vi "Set Mode.vi"(8 "error in (no error)":errorcluster, 11 "Instrument in":refnum<class "Instrument.lvclass">) -> (0 "error out":errorcluster, 3 "Instrument out":refnum<class "Instrument.lvclass">)   [LabVIEW 2018, in "Instrument.lvclass"]
uses:
  Instrument.lvclass
  Instrument.lvclass/Instrument.ctl
  Device/Optics/Optics.lvclass/Optics.ctl
  Device/Optics/Opt_Selector/Opt_Selector.lvclass
  C:/Users/devstaff/sparc4/s4gui/Versao ZeroMQ REQ-REP/SPARC4_GUI -20241030/Device/Optics/Optics.lvclass
  Device/Optics/Opt_Continuous/Opt_Continuous.lvclass
  Server/Server.lvclass
  Device/Optics/Optics.lvclass
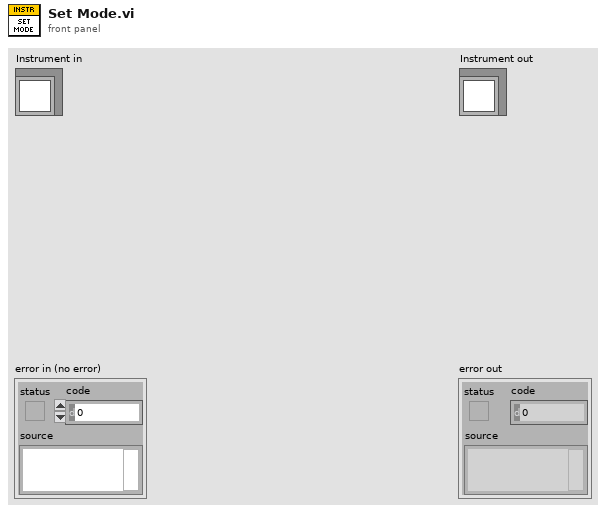
[diagram p1: front panel]
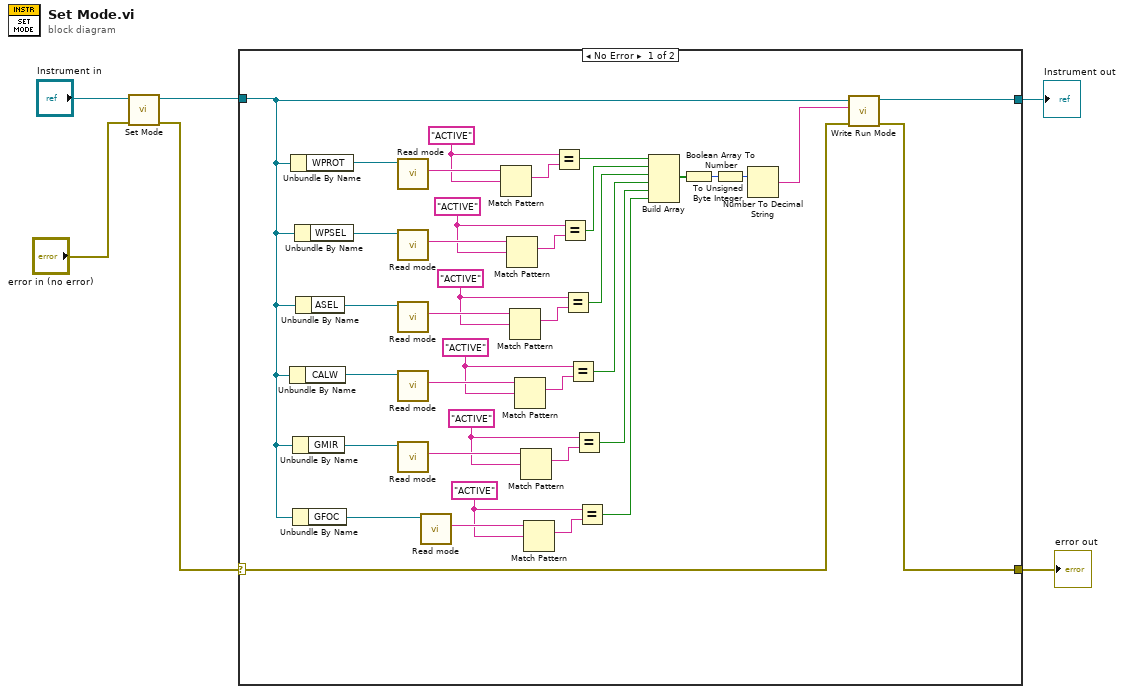
[diagram p0: block diagram]
diagram:
  n1 = call-parent "Set Mode.vi"("error in (no error)"="error in (no error)", "Server in"="Instrument in") -> ("error out"=w4:errorcluster, "Server out"=w3:refnum<class "Instrument.lvclass">)  [unwired: 8 in]
  n2 = case shown="No Error" w4 {
    selector: w4 -> [w18 w45]
    tunnel: w3 -> [w20 w46]
    tunnel: [w19 w46] -> w2
    tunnel: [w17 w45] -> w1
    frame No Error {
      w22 = "ACTIVE"
      w26 = "ACTIVE"
      w29 = "ACTIVE"
      w34 = "ACTIVE"
      w38 = "ACTIVE"
      w41 = "ACTIVE"
      n3 = Unbundle By Name(w20) -> ("CALW"=w32:refnum<class "Opt_Selector.lvclass">)
      n4 = Unbundle By Name(w20) -> ("WPROT"=w44:refnum<class "Opt_Selector.lvclass">)
      n5 = Unbundle By Name(w20) -> ("GMIR"=w25:refnum<class "Opt_Continuous.lvclass">)
      n6 = Unbundle By Name(w20) -> ("GFOC"=w21:refnum<class "Opt_Continuous.lvclass">)
      n7 = Unbundle By Name(w20) -> ("WPSEL"=w37:refnum<class "Opt_Selector.lvclass">)
      n8 = Unbundle By Name(w20) -> ("ASEL"=w33:refnum<class "Opt_Selector.lvclass">)
      n9 = call "Read mode.vi"("Optics in"=w44) -> ("mode"=w43:string)  [unwired: 8 in, 2 out]
      n10 = call "Read mode.vi"("Optics in"=w37) -> ("mode"=w40:string)  [unwired: 8 in, 2 out]
      n11 = call "Read mode.vi"("Optics in"=w33) -> ("mode"=w36:string)  [unwired: 8 in, 2 out]
      n12 = call "Read mode.vi"("Optics in"=w32) -> ("mode"=w31:string)  [unwired: 8 in, 2 out]
      n13 = call "Read mode.vi"("Optics in"=w25) -> ("mode"=w28:string)  [unwired: 8 in, 2 out]
      n14 = call "Read mode.vi"("Optics in"=w21) -> ("mode"=w24:string)  [unwired: 8 in, 2 out]
      n15 = Match Pattern(string=w43, regular expression=w41) -> (match substring=w42:string)  [unwired: 1 in, 3 out]
      n16 = Match Pattern(string=w40, regular expression=w38) -> (match substring=w39:string)  [unwired: 1 in, 3 out]
      n17 = Match Pattern(string=w36, regular expression=w34) -> (match substring=w35:string)  [unwired: 1 in, 3 out]
      n18 = Match Pattern(string=w31, regular expression=w29) -> (match substring=w30:string)  [unwired: 1 in, 3 out]
      n19 = Match Pattern(string=w28, regular expression=w26) -> (match substring=w27:string)  [unwired: 1 in, 3 out]
      n20 = Match Pattern(string=w24, regular expression=w22) -> (match substring=w23:string)  [unwired: 1 in, 3 out]
      n21 = Equal?(x=w41, y=w42) -> (x = y?=w16:bool)
      n22 = Equal?(x=w38, y=w39) -> (x = y?=w15:bool)
      n23 = Equal?(x=w34, y=w35) -> (x = y?=w14:bool)
      n24 = Equal?(x=w29, y=w30) -> (x = y?=w13:bool)
      n25 = Equal?(x=w26, y=w27) -> (x = y?=w12:bool)
      n26 = Equal?(x=w22, y=w23) -> (x = y?=w11:bool)
      n27 = Build Array(w16, w15, w14, w13, w12, w11) -> (w10:bool[])
      n28 = Boolean Array To Number(Boolean array=w10) -> (number=w9:u32)
      n29 = To Unsigned Byte Integer(number=w9) -> (unsigned 8bit integer=w7:u8)
      n30 = Number To Decimal String(number=w7) -> (decimal integer string=w8:string)  [unwired: 1 in]
      n31 = call-dynamic "Write Run Mode.vi"("error in (no error)"=w18, "Run Mode"=w8, "Server in"=w20) -> ("error out"=w17:errorcluster, "Server out"=w19:refnum<class "Instrument.lvclass">)  [unwired: 7 in]
    }
    frame Error {
    }
  }
  "error out" <- w1
  "Instrument out" <- w2
